vi "SysTest-Config.vi"(0 "AO Control":T2[](xcontrol), 1 "Waveform Graph":refnum<vi>, 2 "Data Folder":path, 3 "Trigger":bool, 5 "Item Symbols":i32[](array[numeric]), 7 "AO Chans":i32[](array[numeric]), 9 "AI Chans":i32[](array[numeric]), 11 "error in (no error)":errorcluster, 12 "AO Sampling Rate (Hz)":dbl, 13 "AI Sampling Rate (Hz)":dbl, 14 "Total Duration (ms)":dbl) -> (4 "have AI?":bool, 6 "StimChans Out":T1 {"Filter"."Stages"."IIR Filter"."Forward Coefficients" format="%.4f"; "Filter"."Stages"."IIR Filter"."Reverse Coefficients" format="%.4f"}, 8 "AO npts":i32, 10 "AO Chans":i32[](array[numeric]), 15 "error out":errorcluster)   [LabVIEW 2020]
uses:
  epl-vi-lib/PXI DAQ VIs/DAQ Engine VIs/PXI Globals.vi
  epl-vi-lib/Utility VIs/Type Defs/Speaker ring.ctl
  epl-vi-lib/Signal Synthesis VIs/Controls/Multichannel (Full)/Multichannel (Full).xctl
  epl-vi-lib/Signal Synthesis VIs/Filter VIs/Filter-Bandwidth Units.ctl
  epl-vi-lib/Signal Synthesis VIs/Controls/Advanced Filter XCtl/Filter Data.ctl
  epl-vi-lib/Signal Synthesis VIs/Controls/Advanced Filter XCtl/Advanced Filter XCtl.xctl
  epl-vi-lib/Signal Synthesis VIs/Controls/Level XCtl/Level Units.ctl
  epl-vi-lib/Signal Synthesis VIs/Controls/Level XCtl/Level Data.ctl
  epl-vi-lib/Signal Synthesis VIs/Controls/Level XCtl/Level XCtl.xctl
  epl-vi-lib/Signal Synthesis VIs/Controls/Burst XCtl/Burst Data.ctl
  epl-vi-lib/Signal Synthesis VIs/Controls/Burst XCtl/Burst Control.xctl
  epl-vi-lib/Signal Synthesis VIs/Controls/Waveform XCtl/Waveform Enum.ctl
  epl-vi-lib/Signal Synthesis VIs/Waveform VIs/Tone VIs/Tone Params.ctl
  epl-vi-lib/Signal Synthesis VIs/Waveform VIs/Pulse Train VIs/Pulse Polarity.ctl
  epl-vi-lib/Signal Synthesis VIs/Waveform VIs/Pulse Train VIs/PT-Continuous State.ctl
  epl-vi-lib/Signal Synthesis VIs/Waveform VIs/Pulse Train VIs/Pulse Train Params.ctl
  epl-vi-lib/Signal Synthesis VIs/Waveform VIs/Noise VIs/Noise Params.ctl
  epl-vi-lib/Signal Synthesis VIs/Waveform VIs/File VIs/StimFile-Params.ctl
  epl-vi-lib/Signal Synthesis VIs/Waveform VIs/FM Sweep VIs/FM Sweep Params.ctl
  epl-vi-lib/Signal Synthesis VIs/Waveform VIs/Chirp Train VIs/Chirp Train Params.ctl
  epl-vi-lib/Signal Synthesis VIs/Waveform VIs/Chirp Train VIs/Chirp Train.ctl
  epl-vi-lib/Signal Synthesis VIs/Waveform VIs/Complex Tone VIs/CT-Phase Enum.ctl
  epl-vi-lib/Signal Synthesis VIs/Waveform VIs/Complex Tone VIs/CT-Params.ctl
  epl-vi-lib/Signal Synthesis VIs/Waveform VIs/Complex Tone VIs/CT-Runtime Data.ctl
  epl-vi-lib/Signal Synthesis VIs/Controls/Waveform XCtl/Waveform Data.ctl
  epl-vi-lib/Signal Synthesis VIs/Controls/Waveform XCtl/Waveform XCtl.xctl
  epl-vi-lib/Signal Synthesis VIs/Controls/Advanced Options XCtl/Advanced Stimulus Options.ctl
  epl-vi-lib/Signal Synthesis VIs/Controls/Advanced Options XCtl/Advanced Stimulus Options.xctl
  epl-vi-lib/Signal Synthesis VIs/Modulation VIs/SAM VIs/SAM Params.ctl
  epl-vi-lib/Signal Synthesis VIs/Controls/Stimulus Channel (Full)/Full Stimulus Channel Data.ctl
  epl-vi-lib/Signal Synthesis VIs/Controls/Stimulus Channel (Full)/Stimulus Channel (Full).xctl
  epl-vi-lib/Signal Synthesis VIs/Controls/Multichannel (Full)/Data.ctl
  epl-vi-lib/Signal Synthesis VIs/Waveform VIs/Moving Ripple VIs/Moving Ripple.Params.ctl
  epl-vi-lib/Signal Synthesis VIs/Waveform VIs/Moving Ripple VIs/Moving Ripple.Data.ctl
  epl-vi-lib/Signal Synthesis VIs/Waveform VIs/Moving Ripple VIs/Moving Ripple.ctl
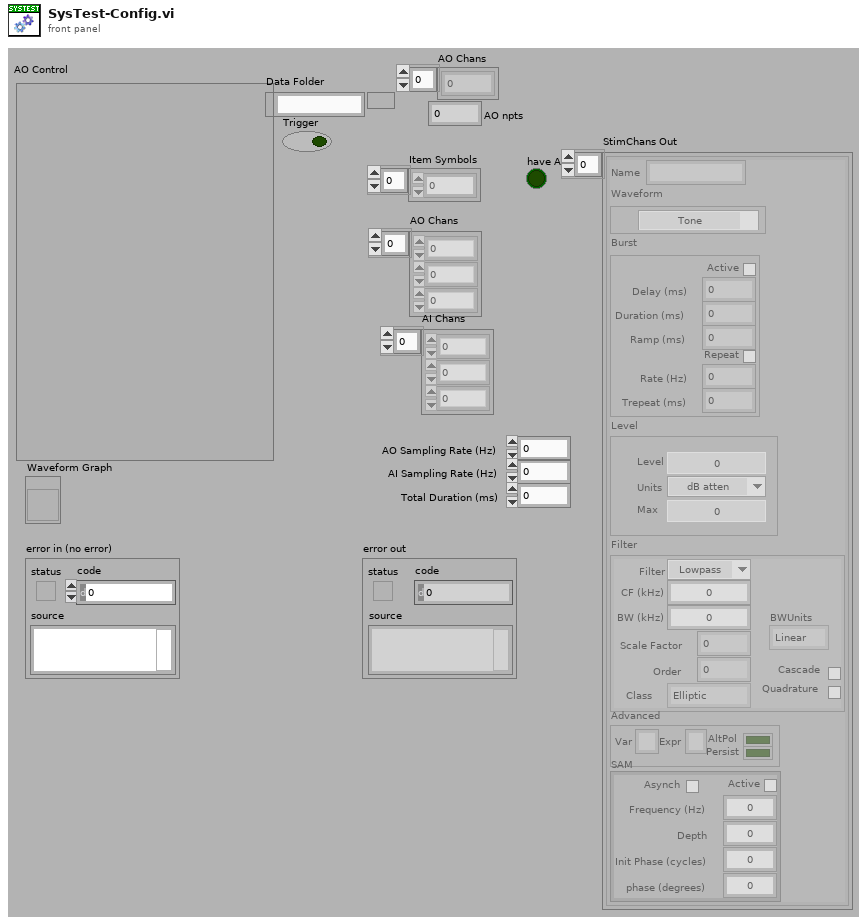
[diagram p1: front panel]
types:
  T1 = typedef "Multichannel (Full).xctl/Data.ctl" = T2[]
  T2 = typedef "Stimulus Channel (Full).xctl/Full Stimulus Channel Data.ctl" = cluster{"Waveform":T3, "Filter":T20, "Burst":T22, "Level":T23, "Name":string, "Advanced":T25, "SAM":T26}
  T3 = typedef "Waveform XCtl.xctl/Waveform Data.ctl" = cluster{"Type":T4, "Tone":T5, "Pulse Train":T6, "Noise":T9, "File":T10, "FMSweep":T11, "Chirp Train":T12, "Complex Tone":cluster{"Params":T14, "Data":T16}, "Moving Ripple":T17}
  T4 = typedef "Waveform Enum.ctl" = enum16{"OFF", "Tone", "Noise", "Pulse Train", "File", "FM Sweep", "Chirp Train", "Complex Tone", "FM Tone", "Moving Ripple"}
  T5 = typedef "Tone Params.ctl" = cluster{"Frequency (kHz)":dbl, "Last Freq":dbl, "Last Phase":dbl}
  T6 = typedef "Pulse Train Params.ctl" = cluster{"Pulse width (us)":dbl, "Pulse rate (Hz)":dbl, "Gap (ms)":dbl, "Polarity":T7, "PT State":T8, "Asynch":bool}
  T7 = typedef "Pulse Polarity.ctl" = enum16{"POS", "NEG", "POS-NEG", "NEG-POS"}
  T8 = typedef "PT-Continuous State.ctl" = cluster{"Template":dbl[], "Nperiod":i32, "Index":i32, "Pulse Rate (Hz)":dbl, "Phase (cycles)":dbl, "Noff":i32}
  T9 = typedef "Noise Params.ctl" = cluster{"InvFilt":bool, "Noise":dbl[], "CurPt":i32, "Aweight":bool, "Seed":i32, "afile":path}
  T10 = typedef "StimFile-Params.ctl" = cluster{"Filename":path, "Signal":dbl[], "Channel":i32, "stream":bool, "offset":i32, "nreps":i32, "loops":i32, "Randomize":bool, "order":i32[], "Seed":i32, "Tokens":i32}
  T11 = typedef "FM Sweep Params.ctl" = cluster{"Rate (oct/s)":dbl, "Fmin (Hz)":dbl, "Fmax (Hz)":dbl, "Ramp (ms)":dbl, "Linear":bool}
  T12 = typedef "Chirp Train.ctl" = cluster{"Params":T13, "Data":cluster{"WF":dbl[]}}
  T13 = typedef "Chirp Train Params.ctl" = cluster{"Fmin (kHz)":dbl, "Fmax (kHz)":dbl, "Compensate":bool, "Duration (ms)":dbl}
  T14 = typedef "CT-Params.ctl" = cluster{"F0 (Hz)":dbl, "Band":cluster{"Flow (Hz)":dbl, "Fhigh (Hz)":dbl}, "Phase":T15, "Min F0 (Hz)":dbl, "Max F0 (Hz)":dbl, "ContinRandPhase":bool, "Max peak factor":dbl, "Max mod depth":dbl, "MinHarmNum":i32, "MaxHarmNum":i32, "Level Mode":enum16{"per component", "overall rms"}, "% jitter":dbl}
  T15 = typedef "CT-Phase Enum.ctl" = enum16{"Cosine", "Random", "Alternating"}
  T16 = typedef "CT-Runtime Data.ctl" = cluster{"Ncomp":i32, "MinHarm":i32, "Phase":dbl[], "Amplitude":dbl[], "Npts/frame":i32, "Last F0":dbl, "Fmin":dbl, "Fmax":dbl, "Lslope":dbl, "randphase":bool, "overall rms":bool, "fmult":dbl[], "jittered":bool}
  T17 = typedef "Moving Ripple.ctl" = cluster{"Params":T18, "Data":T19}
  T18 = typedef "Moving Ripple.Params.ctl" = cluster{"Fmin":dbl, "Fmax":dbl, "Density":dbl, "Velocity":dbl, "Depth":dbl, "Phase":dbl, "Comp/oct":i32}
  T19 = typedef "Moving Ripple.Data.ctl" = cluster{"Freq":dbl[], "A":dbl[], "phase":dbl[], "Phase":dbl}
  T20 = typedef "Advanced Filter XCtl.xctl/Filter Data.ctl" = cluster{"Type":enum16{"Lowpass", "Highpass", "Bandpass", "Bandstop", "OFF"}, "CF (kHz)":dbl, "BW (kHz)":dbl, "Cascade":bool, "Quadrature":bool, "Scale Factor":dbl, "Stages":cluster{"IIR Filter":cluster{"filter structure":enum32{"IIR 2nd Order", "IIR 4th Order"}, "Reverse Coefficients":dbl[], "Forward Coefficients":dbl[]}, "State":dbl[]}[], "Class":enum16{"Elliptic", "Butterworth"}, "Order":i32, "BWUnits":T21}
  T21 = typedef "Filter-Bandwidth Units.ctl" = enum16{"Linear", "Octaves", "Min-Max"}
  T22 = typedef "Burst Control.xctl/Burst Data.ctl" = cluster{"Active":bool, "Delay (ms)":dbl, "Duration (ms)":dbl, "Ramp (ms)":dbl, "Rate (Hz)":dbl, "Trepeat (ms)":dbl, "Repeat":bool}
  T23 = typedef "Level XCtl.xctl/Level Data.ctl" = cluster{"Level":dbl, "Units":T24, "Max":dbl, "Multiplier":dbl, "Cal File":path, "Cal":cluster{"Freq (Hz)":dbl[], "Mag (dB SPL)":dbl[], "Phase (deg)":dbl[]}}
  T24 = typedef "Level Units.ctl" = enum16{"dB atten", "dB SPL", "dB re 1 Vrms", "dB V/Hz½", "mW", "dB HL", "Volts", "dB mW"}
  T25 = typedef "Advanced Stimulus Options.xctl/Advanced Stimulus Options.ctl" = cluster{"Rep Mask":string, "AltPol":bool, "Var":string, "Expr":string, "Persist":bool}
  T26 = typedef "SAM Params.ctl" = cluster{"Active":bool, "Frequency (Hz)":dbl, "Depth":dbl, "Init Phase (cycles)":dbl, "phase (degrees)":dbl, "Asynch":bool}
  T27 = enum16{"Init", "Write", "Read", "Latch setup", "Compute comp.", "Read 1 Channel"}
  T28 = typedef "Speaker ring.ctl" = enum16{"Right primary", "Right secondary", "Left primary", "Left secondary"}
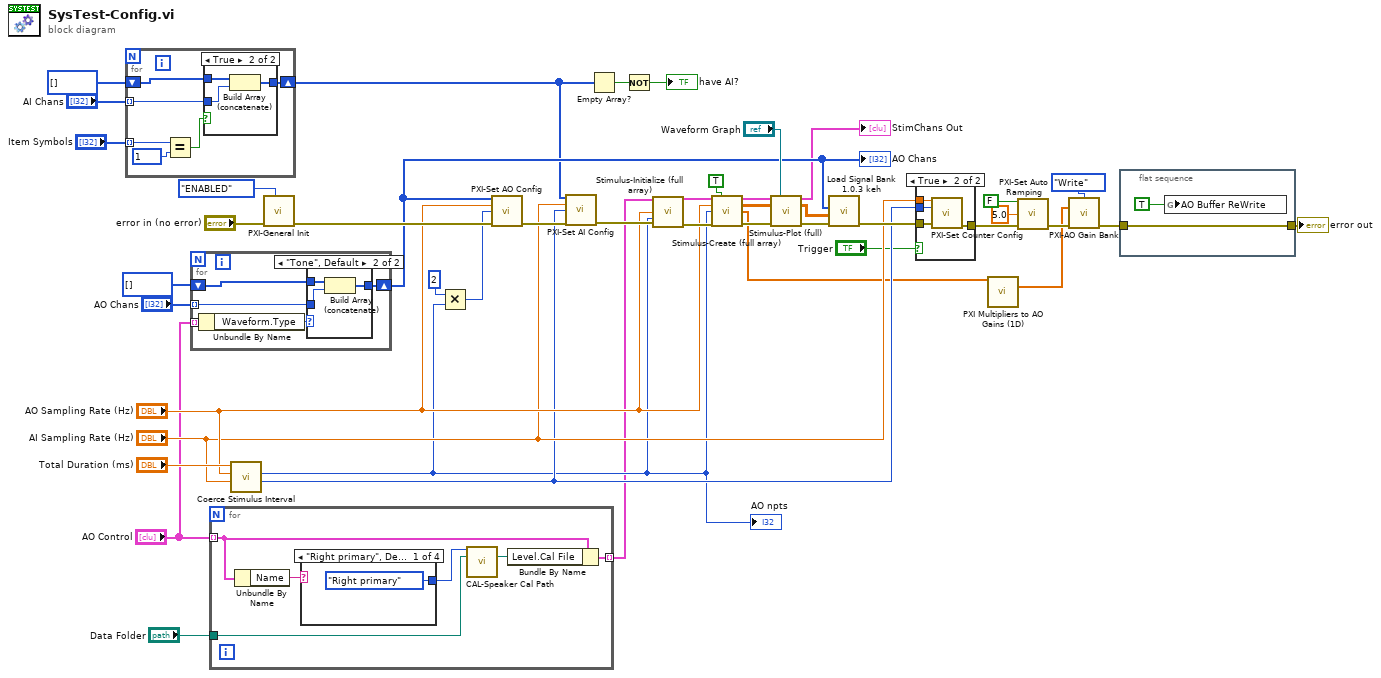
[diagram p0: block diagram]
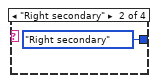
[diagram p3: hidden frame]
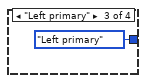
[diagram p4: hidden frame]
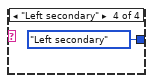
[diagram p5: hidden frame]
diagram:
  n1 = for {
    tunnel: "AI Chans" -> [w51] mode=indexing
    shift-right: [w50] -> w24
    shift-left: i32[] [] -> [w49]
    tunnel: "Item Symbols" -> [w48] mode=indexing
    n2 = Equal?(x=w48, y=1) -> (x = y?=w46:bool)
    n3 = case shown="True" w46 {
      tunnel: w51 -> [_ w55]
      tunnel: [w52 w54] -> w50
      tunnel: w49 -> [w52 w53]
      frame False {
      }
      frame True {
        n4 = Build Array (concatenate)(w53, w55) -> (w54:i32[])
      }
    }
  }
  n5 = for {
    tunnel: "AO Control" -> [w60] mode=indexing
    tunnel: "AO Chans" -> [w58] mode=indexing
    shift-right: [w57] -> w28
    shift-left: i32[] [] -> [w56]
    n6 = Unbundle By Name(w60) -> ("Waveform.Type"=w59:T4)
    n7 = case shown="\"Tone\", Default" w59 {
      tunnel: w58 -> [_ w64]
      tunnel: [w61 w63] -> w57
      tunnel: w56 -> [w61 w62]
      frame "OFF" {
      }
      frame "Tone", Default {
        n8 = Build Array (concatenate)(w62, w64) -> (w63:i32[])
      }
    }
  }
  "AO Chans" <- w28
  n9 = for {
    tunnel: "AO Control" -> [w70] mode=indexing
    tunnel: "Data Folder" -> [w65]
    tunnel: [w69] -> w9 mode=indexing
    n10 = Unbundle By Name(w70) -> ("Name"=w68:string)
    n11 = case shown="\"Right primary\", Default" w68 {
      tunnel: [Speaker_ring."Right primary" ("Speaker") Speaker_ring."Right secondary" ("Speaker") Speaker_ring."Left primary" ("Speaker") Speaker_ring."Left secondary" ("Speaker")] -> w66
      frame "Right primary", Default {
      }
      frame "Right secondary" {
      }
      frame "Left primary" {
      }
      frame "Left secondary" {
      }
    }
    n12 = call "CAL-Speaker Cal Path.vi"("Speaker"=w66, "Data Folder"=w65) -> ("Cal Path"=w67:path)  [unwired: 12 in, 1 out]
    n13 = Bundle By Name(cluster=w70, "Level.Cal File"=w67) -> (w69:T2)
  }
  n14 = call "Coerce Stimulus Interval.vi"("AI sampling rate (Hz)"="AI Sampling Rate (Hz)", "AO sampling rate (Hz)"="AO Sampling Rate (Hz)", "Stimulus interval (ms)"="Total Duration (ms)") -> ("AI npts"=w18:i32, "AO npts"=w15:i32)  [unwired: 5 in, 2 out]
  "AO npts" <- w15
  n15 = call "PXI-General Init.vi"("Double Buffer Mode"=enum32{"OFF", "ENABLED", "FORCED"}."ENABLED", "error in (no error)"="error in (no error)") -> ("error out"=w44:errorcluster)  [unwired: 9 in]
  n16 = Multiply(x=2, y=w15) -> (x*y=w26:i32)
  n17 = call "PXI-Set AO Config.vi"("AO Channels"=w28, "Sampling Rate (Hz)"="AO Sampling Rate (Hz)", "Buffer Size"=w26, "error in (no error)"=w44) -> ("error out"=w25:errorcluster)  [unwired: 11 in]
  n18 = call "PXI-Set AI Config.vi"("AI Channels"=w24, "Sampling Rate (Hz)"="AI Sampling Rate (Hz)", "Buffer Size"=w18, "error in (no error)"=w25) -> ("error out"=w45:errorcluster)  [unwired: 11 in]
  n19 = Empty Array?(array=w24) -> (empty?=w23:bool)
  n20 = Not(x=w23) -> (.not. x?=→"have AI?":bool)
  n21 = call "Stimulus-Initialize (full array).vi"("StimChans"=w9, "Sampling rate (Hz)"="AO Sampling Rate (Hz)", "Npts"=w15, "error in (no error)"=w45) -> ("StimChans Out"=w29:T2[], "error out"=w30:errorcluster)  [unwired: 9 in, 1 out]
  n22 = call "Stimulus-Create (full array).vi"("StimChan"=w29, "Apply multipliers? (F)"=TRUE ("Apply multipliers?"), "Sampling Rate (Hz)"="AO Sampling Rate (Hz)", "Npts"=w15, "error in (no error)"=w30) -> ("StimChan Out"=w33:T2[], "Waveform"=w7:dbl[][], "Multipliers"=w6:dbl[], "error out"=w35:errorcluster)  [unwired: 7 in]
  n23 = call "Stimulus-Plot (full).vi"("AO Control"=w33, "Waveform Graph"="Waveform Graph", "Array"=w7, "error in (no error)"=w35) -> ("AO Control out"=→"StimChans Out":T2[], "Array out"=w21:dbl[][], "error out"=w34:errorcluster)  [unwired: 9 in]
  n24 = call "Load Signal Bank 1.0.3 keh.vi"("error in (no error)"=w34, "Input array"=w21, "Active AO Array"=w28) -> ("error out"=w20:errorcluster)  [unwired: 6 in, 2 out]
  n25 = case shown="True" "Trigger" {
    tunnel: w20 -> [w75 w79]
    tunnel: "AI Sampling Rate (Hz)" -> [_ w78]
    tunnel: w18 -> [_ w77]
    tunnel: [w75 w76] -> w14
    frame False {
    }
    frame True {
      n26 = call "PXI-Set Counter Config.vi"("AI Sampling Rate (Hz)"=w78, "Num AI Pts"=w77, "error in (no error)"=w79) -> ("error out"=w76:errorcluster)  [unwired: 12 in]
    }
  }
  n27 = call "PXI Multipliers to AO Gains (1D).vi"("Multipliers in"=w6) -> ("Gains"=w2:dbl[])  [unwired: 12 in, 2 out]
  n28 = call "PXI-Set Auto Ramping.vi"("Auto ramp?"=FALSE, "Ramp duration (ms)"=5.0, "error in (no error)"=w14) -> ("error out"=w4:errorcluster)  [unwired: 12 in]
  n29 = call "PXI-AO Gain Bank.vi"("Action"=T27."Write", "Gains"=w2, "error in (no error)"=w4) -> ("error out"=w3:errorcluster)  [unwired: 7 in, 5 out]
  n30 = flat-sequence {
    tunnel: w3 -> [w81]
    tunnel: [w81] -> w17
    frame #0 {
      n31 = global write "PXI Globals.vi" "AO Buffer ReWrite"(TRUE ("AO Buffer ReWrite")) -> ()
    }
  }
  "error out" <- w17
